vi "enum.vi"() -> ()   [LabVIEW 2020]
panel:
  out "Waveform Graph 9":dbl[](graph)
  out "Waveform Graph 8":dbl[](graph)
  out "Waveform Graph 7":dbl[](graph)
  out "Waveform Graph 6":dbl[](graph)
  out "Waveform Graph 5":dbl[](graph)
  out "Waveform Graph 4":dbl[](graph)
  out "Waveform Graph 3":dbl[](graph)
  out "Waveform Graph 2":dbl[](graph)
  out "Waveform Graph":dbl[](graph)
  in  "Enum":enum16{"tansec", "cotcosec", "sincos"}(ring)
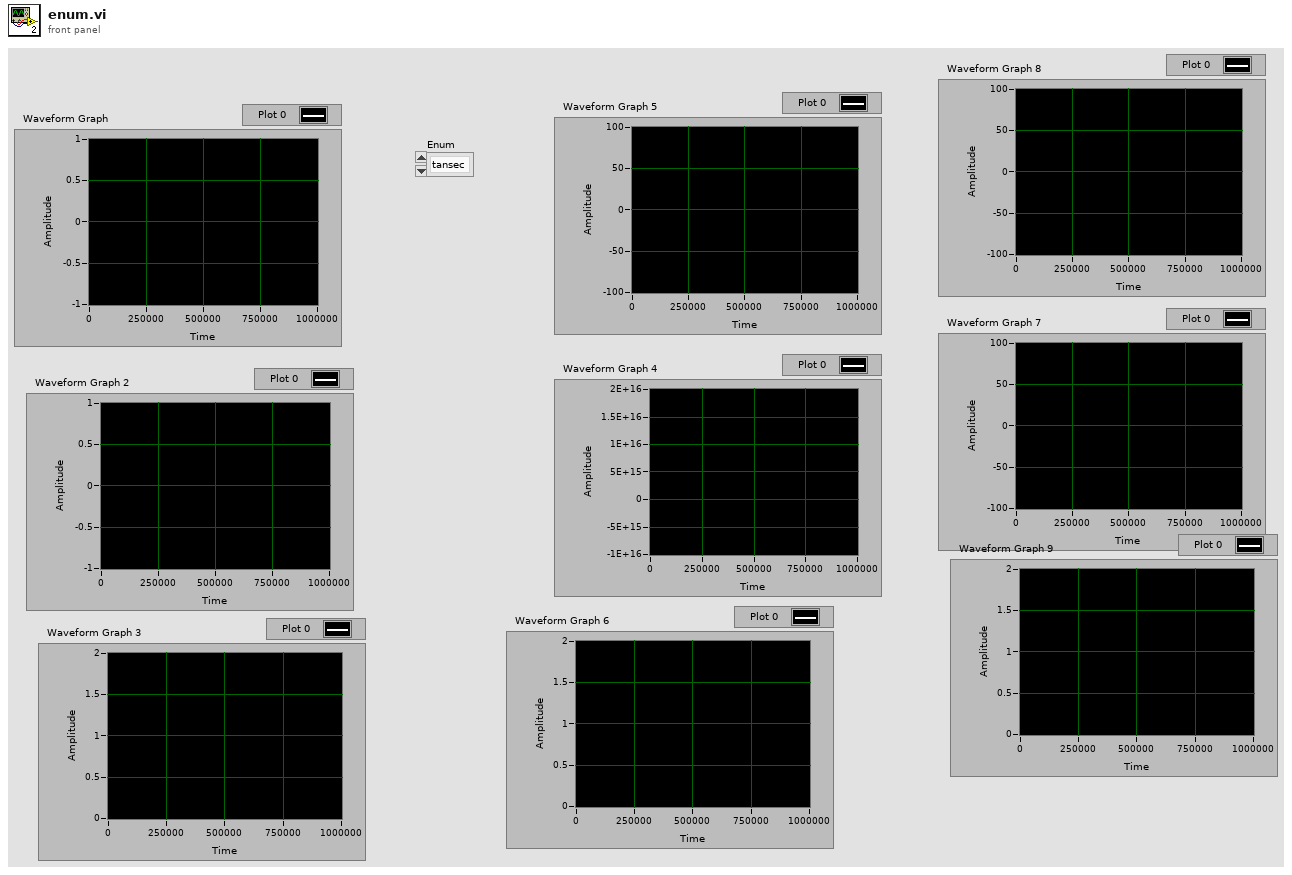
[diagram p1: front panel]
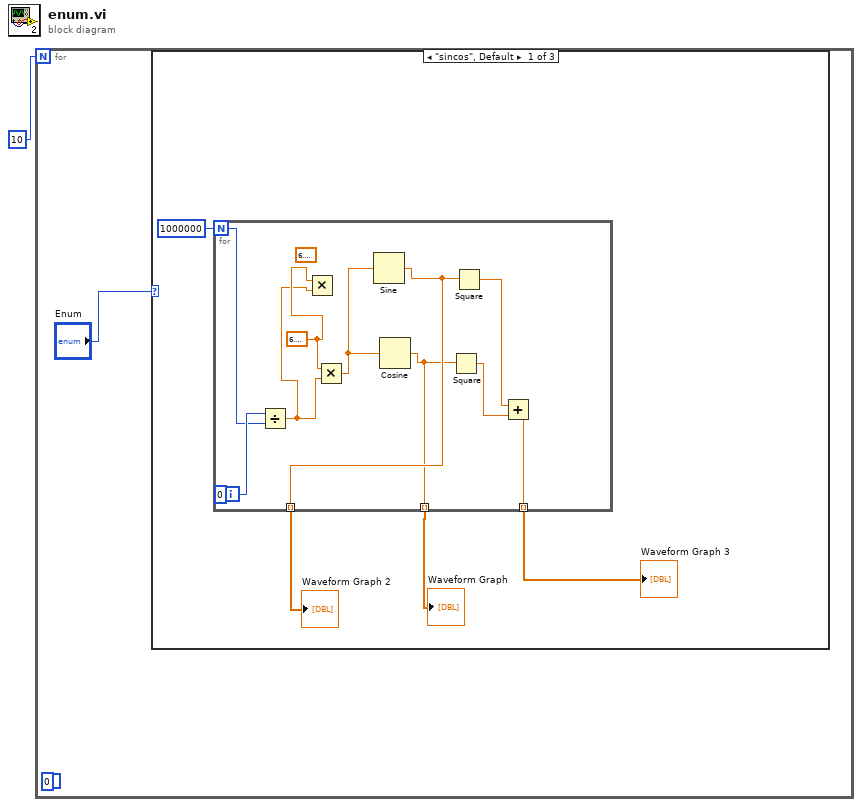
[diagram p0: block diagram]
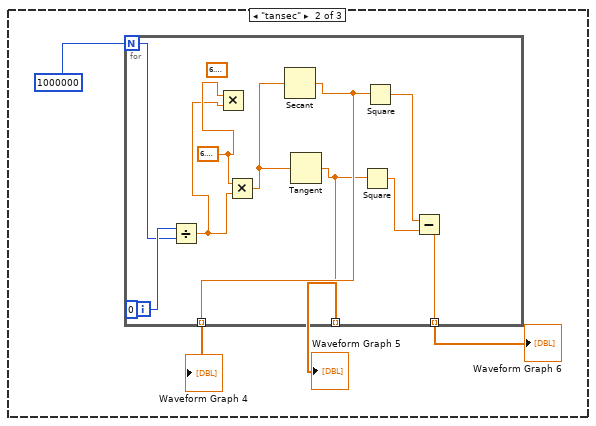
[diagram p2: hidden frame]
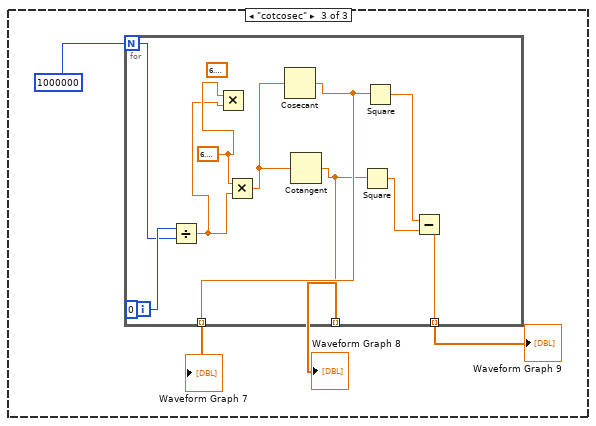
[diagram p3: hidden frame]
diagram:
  n1 = for {
    N: 10 -> [_]
    (unwired) 0
    n2 = case shown="\"sincos\", Default" "Enum" {
      frame "sincos", Default {
        n3 = for {
          N: 1000000 -> [w15]
          tunnel: [w9] -> w5 mode=indexing
          tunnel: [w8] -> w4 mode=indexing
          tunnel: [w7] -> w3 mode=indexing
          i -> [w16]
          (unwired) 0
          w14 = 6.283185307179586
          (unwired) 6.283185307179586
          n4 = Divide(x=w16, y=w15) -> (x/y=w10:dbl)
          n5 = Multiply(x=w14, y=w10) -> ()  [unwired: 1 out]
          n6 = Multiply(x=w14, y=w10) -> (x*y=w13:dbl)
          n7 = Sine(x=w13) -> (sin(x)=w9:dbl)
          n8 = Cosine(x=w13) -> (cos(x)=w8:dbl)
          n9 = Square(x=w8) -> (x^2=w11:dbl)
          n10 = Square(x=w9) -> (x^2=w12:dbl)
          n11 = Add(x=w12, y=w11) -> (x+y=w7:dbl)
        }
        "Waveform Graph 2" <- w5
        "Waveform Graph" <- w4
        "Waveform Graph 3" <- w3
      }
      frame "tansec" {
        n12 = for {
          N: 1000000 -> [w29]
          tunnel: [w23] -> w19 mode=indexing
          tunnel: [w22] -> w18 mode=indexing
          tunnel: [w21] -> w17 mode=indexing
          i -> [w30]
          (unwired) 0
          w28 = 6.283185307179586
          (unwired) 6.283185307179586
          n13 = Divide(x=w30, y=w29) -> (x/y=w24:dbl)
          n14 = Multiply(x=w28, y=w24) -> ()  [unwired: 1 out]
          n15 = Multiply(x=w28, y=w24) -> (x*y=w27:dbl)
          n16 = Secant(1:w27) -> (0:w23:dbl)
          n17 = Tangent(1:w27) -> (0:w22:dbl)
          n18 = Square(x=w22) -> (x^2=w25:dbl)
          n19 = Square(x=w23) -> (x^2=w26:dbl)
          n20 = Subtract(x=w26, y=w25) -> (x-y=w21:dbl)
        }
        "Waveform Graph 4" <- w19
        "Waveform Graph 5" <- w18
        "Waveform Graph 6" <- w17
      }
      frame "cotcosec" {
        n21 = for {
          N: 1000000 -> [w43]
          tunnel: [w37] -> w33 mode=indexing
          tunnel: [w36] -> w32 mode=indexing
          tunnel: [w35] -> w31 mode=indexing
          i -> [w44]
          (unwired) 0
          w42 = 6.283185307179586
          (unwired) 6.283185307179586
          n22 = Divide(x=w44, y=w43) -> (x/y=w38:dbl)
          n23 = Multiply(x=w42, y=w38) -> ()  [unwired: 1 out]
          n24 = Multiply(x=w42, y=w38) -> (x*y=w41:dbl)
          n25 = Cosecant(1:w41) -> (0:w37:dbl)
          n26 = Cotangent(1:w41) -> (0:w36:dbl)
          n27 = Square(x=w36) -> (x^2=w39:dbl)
          n28 = Square(x=w37) -> (x^2=w40:dbl)
          n29 = Subtract(x=w40, y=w39) -> (x-y=w35:dbl)
        }
        "Waveform Graph 7" <- w33
        "Waveform Graph 8" <- w32
        "Waveform Graph 9" <- w31
      }
    }
  }
